vi "ChangeSetup.vi"(8 "error in":errorcluster, 9 "Targets":T1, 11 "Script":T2[](array[typedef])) -> (0 "error out":errorcluster)   [LabVIEW 2015]
uses:
  Config/Script_actions.ctl
  Systems/Primary Filter/f1driveractions.ctl
  Systems/Secondary Filter/f2driveractions.ctl
  Systems/Coll_Focus/coll_actions.ctl
  Systems/Wavelength/wavelength_parameters.ctl
  Systems/Wavelength/movetypes.ctl
  Systems/Wavelength/wavelength_driver_actions.ctl
  Systems/Grating_Translation/GTdriveractions.ctl
  Systems/Slit/slitactions.ctl
  Systems/Cam_Focus/CF_drivercontrol.ctl
  Systems/Primary Filter/GSP_F1_Global.vi
  Systems/Secondary Filter/GSP_F2_Global.vi
  Systems/Coll_Focus/GSP_COLL_Global.vi
  Systems/Wavelength/GSP_Wavelength_Global.vi
  Systems/Grating_Translation/GSP_GT_Global.vi
  Systems/Slit/GSP_SLIT_Global.vi
  Systems/Cam_Focus/GSP_CF_Global.vi
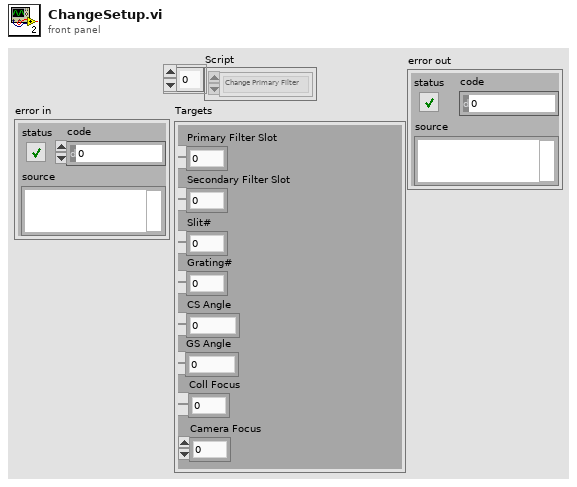
[diagram p1: front panel]
types:
  T1 = cluster{"Primary Filter Slot":i32, "Secondary Filter Slot":i32, "Slit#":i32, "Grating#":i32, "CS Angle":dbl, "GS Angle":dbl, "Coll Focus":i32, "Camera Focus":i32}
  T2 = typedef "Script_actions.ctl" = enum16{"Change Primary Filter", "Change Secondary Filter", "Change Collimator Focus", "Change Camera Focus", "Change Grating", "Change Angles", "Change Slit Mask"}
  T3 = typedef "f1driveractions.ctl" = enum16{"Launch", "INIT_CTL", "Home", "Move", "Shutdown"}
  T4 = typedef "f2driveractions.ctl" = enum16{"Launch", "INIT_CTL", "Home", "Move", "Shutdown"}
  T5 = typedef "coll_actions.ctl" = enum16{"Launch", "Move", "Home", "Open Shutter", "Close Shutter", "Shutdown"}
  T6 = typedef "wavelength_driver_actions.ctl" = enum16{"Launch", "Flexure On", "Flexure Off", "Move", "Home", "Shutdown"}
  T7 = typedef "wavelength_parameters.ctl" = cluster{"Camera Angle":dbl, "Grating  Angle":dbl, "Move type":T8}
  T8 = typedef "movetypes.ctl" = u16
  T9 = typedef "GTdriveractions.ctl" = enum16{"Launch", "INIT_CTL", "Move", "Home", "Shutdown"}
  T10 = typedef "slitactions.ctl" = enum16{"Launch", "INIT_CTL", "Restart", "Show", "Hide", "Home", "Move", "Rotate Only", "Shutdown"}
  T11 = typedef "CF_drivercontrol.ctl" = enum16{"Launch", "Move", "Set Piezos", "Flexure On", "Flexure Off", "Home", "Shutdown"}
  T12 = typedef "ThreadStates.ctl" = enum16{"Waiting", "Scripting", "Uninitialized", "Error"}
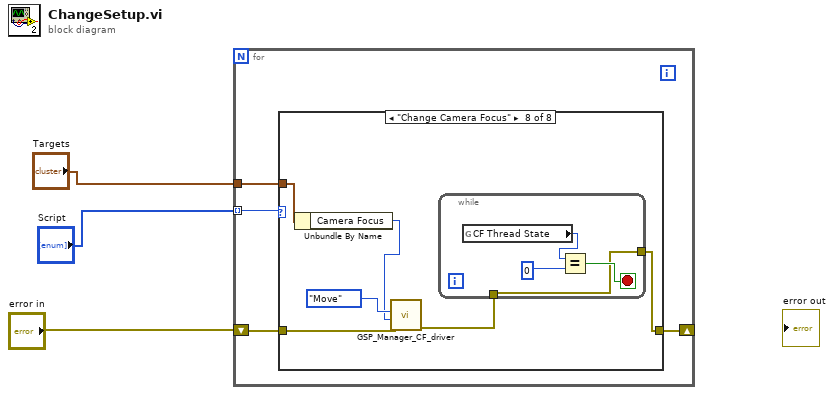
[diagram p0: block diagram]
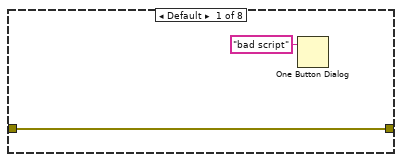
[diagram p2: hidden frame]
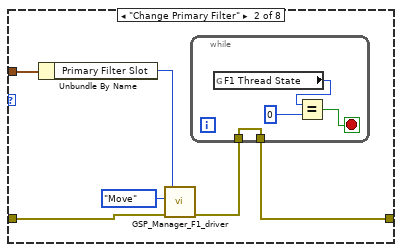
[diagram p3: hidden frame]
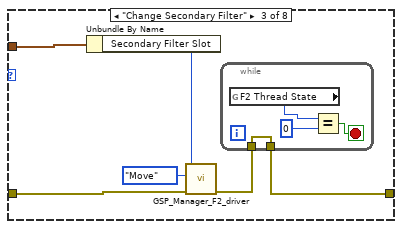
[diagram p4: hidden frame]
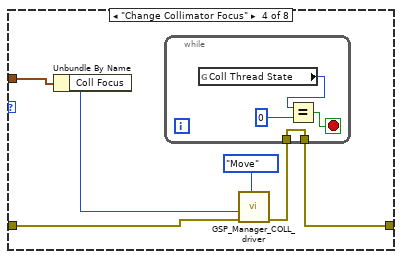
[diagram p5: hidden frame]
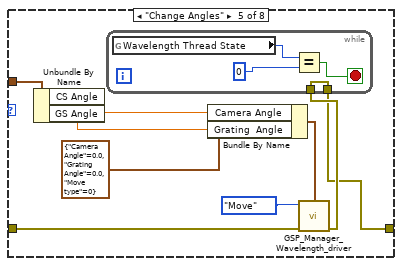
[diagram p6: hidden frame]
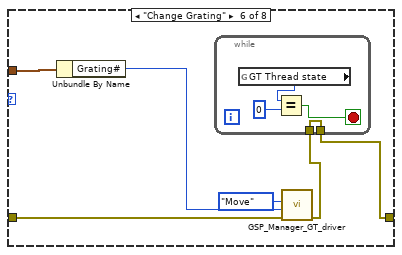
[diagram p7: hidden frame]
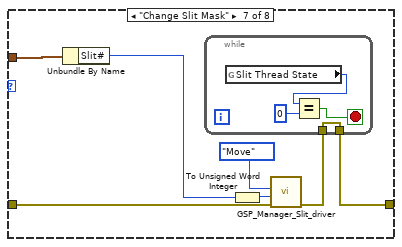
[diagram p8: hidden frame]
diagram:
  n1 = for {
    tunnel: "Script" -> [w6] mode=indexing
    shift-right: [w4] -> _
    shift-left: "error in" -> [w7]
    tunnel: "Targets" -> [w5]
    n2 = case shown="\"Change Camera Focus\"" w6 {
      tunnel: w7 -> [w9 w14 w24 w34 w48 w57 w67 w79]
      tunnel: w5 -> [_ w15 w25 w35 w45 w58 w69 w77]
      tunnel: [w9 w10 w20 w30 w40 w53 w63 w74] -> w4
      frame Default {
        n3 = One Button Dialog(message="bad script") -> ()  [unwired: 1 in, 1 out]
      }
      frame "Change Primary Filter" {
        n4 = Unbundle By Name(w15) -> ("Primary Filter Slot"=w13:i32)
        n5 = call "GSP_Manager_F1_driver.vi"("error in (no error)"=w14, "Action"=f1driveractions."Move", "Filter# (Move Only)"=w13) -> ("error out"=w11:errorcluster)  [unwired: 3 in, 1 out]
        n6 = while {
          tunnel: w11 -> [w16]
          tunnel: [w16] -> w10
          stop <- w17 stop-if-true
          n7 = global read "GSP_F1_Global.vi" "F1 Thread State"() -> (w19:T12)
          n8 = Equal?(x=w19, y=0) -> (x = y?=w17:bool)
        }
      }
      frame "Change Secondary Filter" {
        n9 = Unbundle By Name(w25) -> ("Secondary Filter Slot"=w22:i32)
        n10 = call "GSP_Manager_F2_driver.vi"("error in (no error)"=w24, "Action"=f2driveractions."Move", "Filter# (Move Only)"=w22) -> ("error out"=w21:errorcluster)  [unwired: 3 in, 1 out]
        n11 = while {
          tunnel: w21 -> [w26]
          tunnel: [w26] -> w20
          stop <- w27 stop-if-true
          n12 = global read "GSP_F2_Global.vi" "F2 Thread State"() -> (w28:T12)
          n13 = Equal?(x=w28, y=0) -> (x = y?=w27:bool)
        }
      }
      frame "Change Collimator Focus" {
        n14 = Unbundle By Name(w35) -> ("Coll Focus"=w33:i32)
        n15 = call "GSP_Manager_COLL_driver.vi"("error in (no error)"=w34, "Target (Move Only)"=w33, "Action"=coll_actions."Move") -> ("error out"=w31:errorcluster)  [unwired: 3 in, 1 out]
        n16 = while {
          tunnel: w31 -> [w36]
          tunnel: [w36] -> w30
          stop <- w37 stop-if-true
          n17 = global read "GSP_COLL_Global.vi" "Coll Thread State"() -> (w38:T12)
          n18 = Equal?(x=w38, y=0) -> (x = y?=w37:bool)
        }
      }
      frame "Change Angles" {
        n19 = Unbundle By Name(w45) -> ("CS Angle"=w44:dbl, "GS Angle"=w43:dbl)
        n20 = Bundle By Name(cluster=T7 {"Camera Angle"=0.0, "Grating  Angle"=0.0, "Move type"=0} ("Target (Move Only)"), "Camera Angle"=w44, "Grating  Angle"=w43) -> (w46:T7)
        n21 = call "GSP_Manager_Wavelength_driver.vi"("error in (no error)"=w48, "Target (Move Only)"=w46, "Action"=wavelength_driver_actions."Move") -> ("error out"=w41:errorcluster)  [unwired: 3 in, 1 out]
        n22 = while {
          tunnel: w41 -> [w49]
          tunnel: [w49] -> w40
          stop <- w50 stop-if-true
          n23 = global read "GSP_Wavelength_Global.vi" "Wavelength Thread State"() -> (w52:T12)
          n24 = Equal?(x=w52, y=0) -> (x = y?=w50:bool)
        }
      }
      frame "Change Grating" {
        n25 = Unbundle By Name(w58) -> ("Grating#"=w56:i32)
        n26 = call "GSP_Manager_GT_driver.vi"("error in (no error)"=w57, "Grating # (Move Only)"=w56, "Action"=GTdriveractions."Move") -> ("error out"=w54:errorcluster)  [unwired: 3 in, 1 out]
        n27 = while {
          tunnel: w54 -> [w59]
          tunnel: [w59] -> w53
          stop <- w60 stop-if-true
          n28 = global read "GSP_GT_Global.vi" "GT Thread state"() -> (w61:T12)
          n29 = Equal?(x=w61, y=0) -> (x = y?=w60:bool)
        }
      }
      frame "Change Slit Mask" {
        n30 = Unbundle By Name(w69) -> ("Slit#"=w68:i32)
        n31 = To Unsigned Word Integer(number=w68) -> (unsigned 16bit integer=w65:u16)
        n32 = call "GSP_Manager_Slit_driver.vi"("error in (no error)"=w67, "Slit # (Move/Rotate Only)"=w65, "Action"=slitactions."Move") -> ("error out"=w64:errorcluster)  [unwired: 3 in, 1 out]
        n33 = while {
          tunnel: w64 -> [w70]
          tunnel: [w70] -> w63
          stop <- w71 stop-if-true
          n34 = global read "GSP_SLIT_Global.vi" "Slit Thread State"() -> (w72:T12)
          n35 = Equal?(x=w72, y=0) -> (x = y?=w71:bool)
        }
      }
      frame "Change Camera Focus" {
        n36 = Unbundle By Name(w77) -> ("Camera Focus"=w76:i32)
        n37 = call "GSP_Manager_CF_driver.vi"("error in (no error)"=w79, "Target (Move Only)"=w76, "Action"=CF_drivercontrol."Move") -> ("error out"=w75:errorcluster)  [unwired: 4 in, 1 out]
        n38 = while {
          tunnel: [w80] -> w74
          tunnel: w75 -> [w80]
          stop <- w81 stop-if-true
          n39 = global read "GSP_CF_Global.vi" "CF Thread State"() -> (w83:T12)
          n40 = Equal?(x=w83, y=0) -> (x = y?=w81:bool)
        }
      }
    }
  }
